vi "MicroPulse - sys type decoder (extended msg).vi"(7 "sys type":u32) -> (2 "System Type":T1, 3 "String":string)   [LabVIEW 2026, in "MicroPulse_Driver.lvlib"]
uses:
  MicroPulse_Driver.lvlib
  Public/Data/Datatypes/MP - instrument type.ctl
  <instrlib>/Micropulse/Micropulse.lvlib
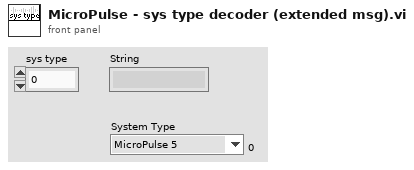
[diagram p1: front panel]
types:
  T1 = typedef "Micropulse.lvlib/MP - instrument type.ctl" = enum16{"MicroPulse 5", "LT1", "LT2", "LTPA", "MPLT", "MicroPulse 6", "PipeScanner", "<MicroPulse>", "Micropulse 4", "Simulated Data"}
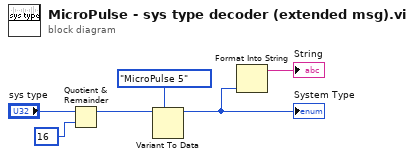
[diagram p0: block diagram]
diagram:
  n1 = Quotient & Remainder(x="sys type", y=u32 16) -> (x-y*floor(x/y)=w2:u32)  [unwired: 1 out]
  n2 = Variant To Data(type=MP_-_instrument_type."MicroPulse 5" ("System Type"), Variant=w2) -> (data=w5:T1)  [unwired: 1 in, 1 out]
  "System Type" <- w5
  n3 = Format Into String(w5) -> (resulting string=→"String":string)  [unwired: 3 in, 1 out]
